vi "generate_waveform.vi"() -> ()   [LabVIEW 2016, in "Utilities.lvlib" / "_TEST.lvlib"]
uses:
  <vilib>/Waveform/DWDTOps.llb/DWDT Analog to Digital.vi
  <vilib>/Waveform/DWDTOps.llb/DWDT Invert Digital.vi
  _TEST.lvlib
  <vilib>/measure/NI_MABase.lvlib
  <vilib>/Analysis/NI_AALBase.lvlib
panel:
  out "scanning frequency (hz)":dbl
  out "sampling frequency (hz)":dbl
  out "daq output":T1(graph)
  out "generated position (v)":dbl[](array[numeric])
  out "generated position (ps)":dbl[](array[numeric])
  out "ideal position (v)":dbl[](array[numeric])
  in  "ratio (v/ps)":dbl
  in  "offset (ps)":dbl
  in  "range (ps)":dbl
  in  "# samples":i32
  in  "gate time (us)":dbl
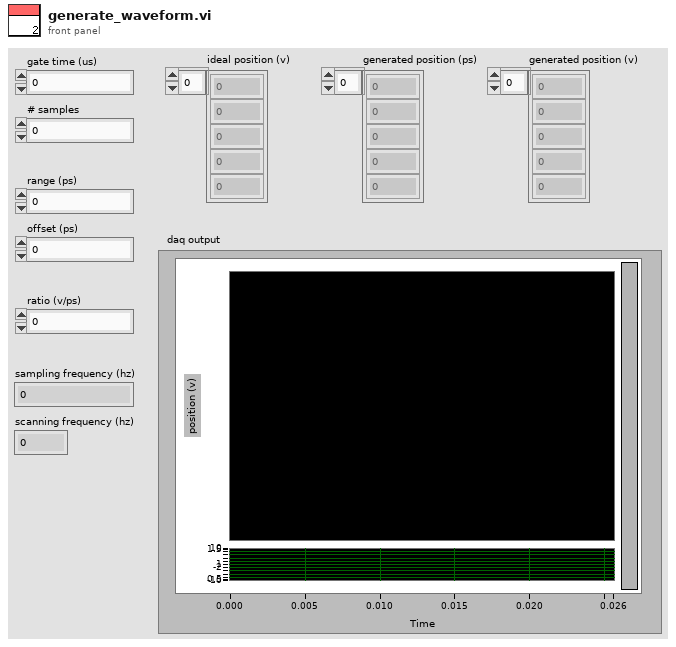
[diagram p1: front panel]
types:
  T1 = cluster{"signal out":waveform(dbl), "digital waveform":digitalwaveform}
  T2 = cluster{"signal out":waveform(dbl), "inverted waveform":digitalwaveform}
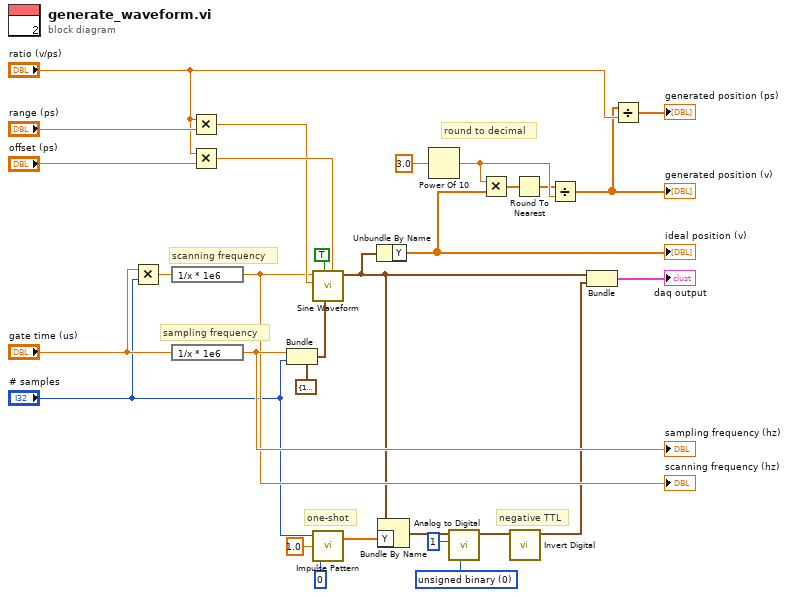
[diagram p0: block diagram]
diagram:
  w3 = u16 0 items=["unsigned binary", "offset binary", "2's complement"] ("data format (offset binary)")
  # "round to decimal"
  # "sampling frequency"
  # "scanning frequency"
  # "one-shot"
  # "negative TTL"
  n1 = Multiply(x="gate time (us)", y="# samples") -> (x*y=w22:dbl)
  n2 = expression code="1/x * 1e6"(w22) -> (w23:dbl)
  "scanning frequency (hz)" <- w23
  n3 = expression code="1/x * 1e6"("gate time (us)") -> (w25:dbl)
  "sampling frequency (hz)" <- w25
  n4 = Multiply(x="ratio (v/ps)", y="range (ps)") -> (x*y=w24:dbl)
  n5 = Multiply(x="ratio (v/ps)", y="offset (ps)") -> (x*y=w26:dbl)
  n6 = Bundle(cluster=cluster{"Fs":dbl, "#s":dbl} {"Fs"=1000.0, "#s"=1000.0} ("sampling info"), "Fs"=w25, "#s"="# samples") -> (w29:cluster{"Fs":dbl, "#s":dbl})
  n7 = call <vilib>:"Sine Waveform.vi"("offset"=w26, "sampling info"=w29, "reset signal"=TRUE, "amplitude"=w24, "frequency"=w23) -> ("signal out"=w6:waveform(dbl))  [unwired: 5 in, 1 out]
  n8 = call <vilib>:"Impulse Pattern.vi"("delay"=0, "amplitude"=1.0, "samples"="# samples") -> ("Impulse Pattern"=w10:dbl[])  [unwired: 1 out]
  n9 = Unbundle By Name(w6) -> ("Y"=w17:dbl[])
  "ideal position (v)" <- w17
  n10 = Bundle By Name(cluster=w6, "Y"=w10) -> (w5:waveform(dbl))
  n11 = Power Of 10(x=3.0) -> (10^x=w13:dbl)
  n12 = call-poly <vilib>:"Analog to Digital.vi"("data format (offset binary)"=w3, "resolution (16 bit)"=1, "analog waveform"=w5) -> ("digital waveform"=w2:digitalwaveform)  [unwired: 5 in, 3 out]
  n13 = Multiply(x=w13, y=w17) -> (x*y=w12:dbl[])
  n14 = call-poly <vilib>:"Invert Digital.vi"("digital waveform"=w2) -> ("inverted waveform"=w1:digitalwaveform)  [unwired: 9 in, 1 out]
  n15 = Round To Nearest(number=w12) -> (nearest integer value=w11:dbl[])
  n16 = Divide(x=w11, y=w13) -> (x/y=w16:dbl[])
  "generated position (v)" <- w16
  n17 = Bundle("signal out"=w6, "inverted waveform"=w1) -> (→"daq output":T2)  [unwired: 1 in]
  n18 = Divide(x=w16, y="ratio (v/ps)") -> (x/y=→"generated position (ps)":dbl[])
